vi "Hold Back Arms (Darius + Allen).vi"(8 "Current Speed":dbl, 9 "Current Height":dbl, 10 "Range":dbl=0.5, 11 "Desired Height":dbl) -> (0 "In Range?":bool)   [LabVIEW 2014]
panel:
  # "starts again from check\nreseting the program"
  # "In inches,from bottom\n(Or any other unit, so long as both are the same"
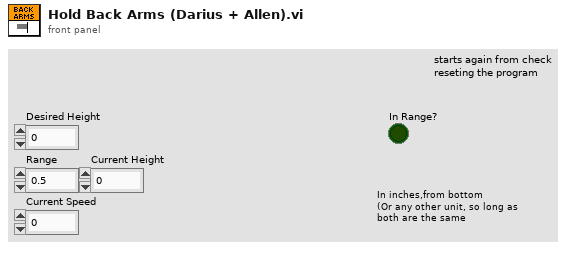
[diagram p1: front panel]
types:
  T1 = typedef "WPI_DigitalInputDevRef.ctl" = cluster{"DevStatus":errorcluster, "DIO Channel":T2, "Controller":T3}
  T2 = typedef "FPGA_DIOChannel.ctl" = enum8{"DIO 0", "DIO 1", "DIO 2", "DIO 3", "DIO 4", "DIO 5", "DIO 6", "DIO 7", "DIO 8", "DIO 9", "DIO MXP 0", "DIO MXP 1", "DIO MXP 2", "DIO MXP 3", "DIO MXP 4", "DIO MXP 5", "DIO MXP 6", "DIO MXP 7", "DIO MXP 8", "DIO MXP 9", "DIO MXP 10", "DIO MXP 11", "DIO MXP 12", "DIO MXP 13", "DIO MXP 14", "DIO MXP 15", "Invalid"}
  T3 = typedef "FPGA_TypedefDigitalModule.ctl" = enum16{"Controller 1"}
  T4 = typedef "WPI_MotorControlDeviceRef.ctl" = cluster{"DeviceStatus":errorcluster, "Type":T5, "PWM":cluster{"Controller":T3, "PWM Channel":T6, "DeadBand":T7}, "CAN":cluster{"Device Number":u8, "Control Mode":T8, "Semaphore":T9, "Max Vout":dbl, "TalonSRX Control Mode":T10}, "Invert":bool, "TransformRef":T11, "InvTransformRef":T11}
  T5 = typedef "WPI_MotorControlType.ctl" = enum16{"PWM", "CAN", "CANTalonSRX"}
  T6 = typedef "FPGA_DIOPWMChannel.ctl" = enum8{"PWM 0", "PWM 1", "PWM 2", "PWM 3", "PWM 4", "PWM 5", "PWM 6", "PWM 7", "PWM 8", "PWM 9", "PWM MXP 0", "PWM MXP 1", "PWM MXP 2", "PWM MXP 3", "PWM MXP 4", "PWM MXP 5", "PWM MXP 6", "PWM MXP 7", "PWM MXP 8", "PWM MXP 9", "Invalid"}
  T7 = typedef "WPI_PWMDeadband.ctl" = cluster{"Name":string, "maxPositivePwm":i32, "minPositivePwm":i32, "centerPwm":i32, "maxNegativePwm":i32, "minNegativePwm":i32, "angularRange":u16}
  T8 = typedef "WPI_CANJaguar_ControlMode.ctl" = enum8{"Percent VBus", "Current", "Speed", "Position", "Voltage"}
  T9 = typedef "Semaphore RefNum" = refnum<k1>
  T10 = typedef "WPI_CANTalonSRX_APIControlMode.ctl" = enum8{"Percent VBus", "Speed", "Position", "Slave", "Unchanged / Invalid"}
  T11 = typedef "WPI_PWMTransform_ConPane.ctl" = refnum<vi>
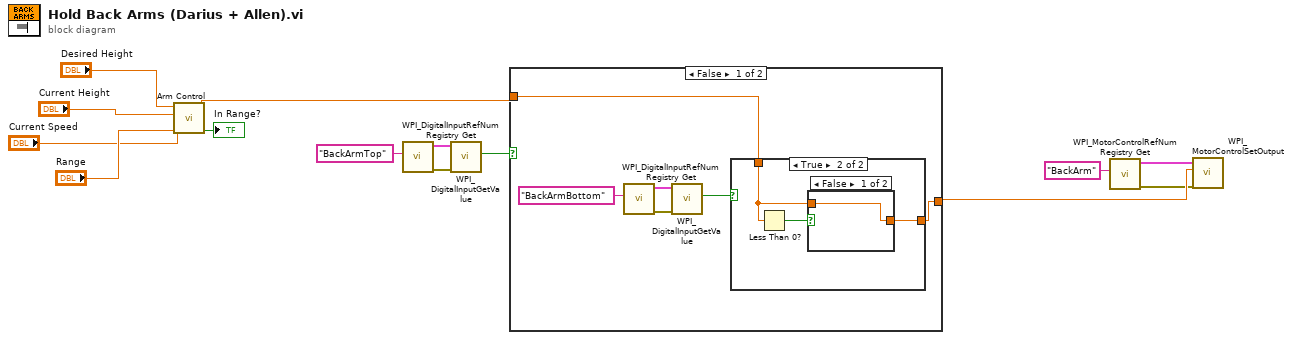
[diagram p0: block diagram]
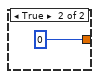
[diagram p3: hidden frame]
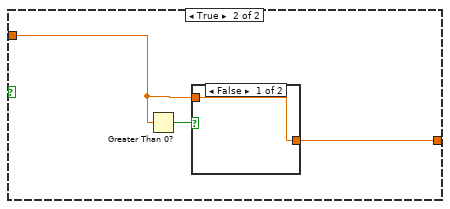
[diagram p4: hidden frame]
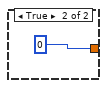
[diagram p5: hidden frame]
diagram:
  n1 = call "Arm Control.vi"("Range"="Range", "Current Speed"="Current Speed", "Current Height"="Current Height", "Desired Height"="Desired Height") -> ("In Range?"=→"In Range?":bool, "Motor Output"=w6:dbl)  [unwired: 6 in]
  n2 = call <vilib>:"WPI_DigitalInputRefNum Registry Get.vi"("refnum name"="BackArmTop") -> ("error out"=w10:errorcluster, "DigitalInputDevRef"=w9:T1)  [unwired: 9 in]
  n3 = call <vilib>:"WPI_DigitalInputGetValue.vi"("error in (no error)"=w10, "DigitalInputDevRef"=w9) -> ("Value"=w7:bool)  [unwired: 7 in, 2 out]
  n4 = case shown="False" w7 {
    tunnel: [w20 w28] -> w14
    tunnel: w6 -> [w15 w27]
    frame False {
      n5 = call <vilib>:"WPI_DigitalInputRefNum Registry Get.vi"("refnum name"="BackArmBottom") -> ("error out"=w19:errorcluster, "DigitalInputDevRef"=w18:T1)  [unwired: 9 in]
      n6 = call <vilib>:"WPI_DigitalInputGetValue.vi"("error in (no error)"=w19, "DigitalInputDevRef"=w18) -> ("Value"=w16:bool)  [unwired: 7 in, 2 out]
      n7 = case shown="True" w16 {
        tunnel: [w21 w23] -> w20
        tunnel: w15 -> [w21 w22]
        frame False {
        }
        frame True {
          n8 = Less Than 0?(x=w22) -> (x < 0?=w24:bool)
          n9 = case shown="False" w24 {
            tunnel: [w25 0] -> w23
            tunnel: w22 -> [w25 _]
            frame False {
            }
            frame True {
            }
          }
        }
      }
    }
    frame True {
      n10 = Greater Than 0?(x=w27) -> (x > 0?=w29:bool)
      n11 = case shown="False" w29 {
        tunnel: [w30 0] -> w28
        tunnel: w27 -> [w30 _]
        frame False {
        }
        frame True {
        }
      }
    }
  }
  n12 = call <vilib>:"WPI_MotorControlRefNum Registry Get.vi"("refnum name"="BackArm") -> ("error out"=w11:errorcluster, "MotorControlDevRef"=w12:T4)  [unwired: 9 in]
  n13 = call <vilib>:"WPI_MotorControlSetOutput.vi"("error in (no error)"=w11, "Output"=w14, "MotorControlDevRef"=w12) -> ()  [unwired: 6 in, 3 out]
